vi "Read Temp (SubVI).vi"(8 "error in (no error)":errorcluster, 10 "Channel":string, 11 "Instrument parameters in in":T1) -> (0 "error out":errorcluster, 2 "Sensor Data":dbl, 3 "Instrument parameters out":T1)   [LabVIEW 2025]
uses:
  TYPE DEFS/S2DS_Instrument parameters.ctl
  Lake Shore 336.lvlib
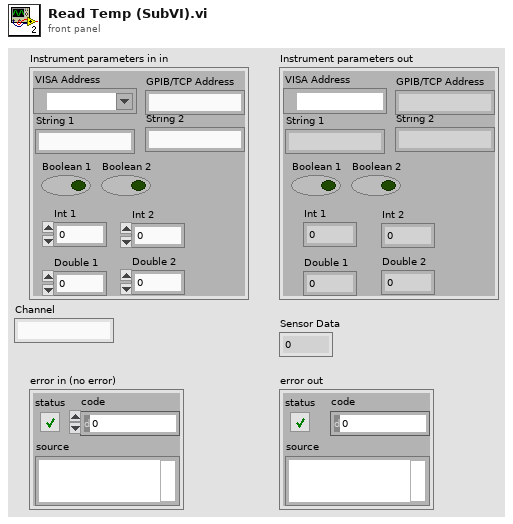
[diagram p1: front panel]
types:
  T1 = typedef "S2DS_Instrument parameters.ctl" = cluster{"VISA Address":refnum<visa-resource-name>, "GPIB/TCP Address":string, "String 1":string, "String 2":string, "Boolean 1":bool, "Boolean 2":bool, "Int 1":i32, "Int 2":i32, "Double 1":dbl, "Double 2":dbl}
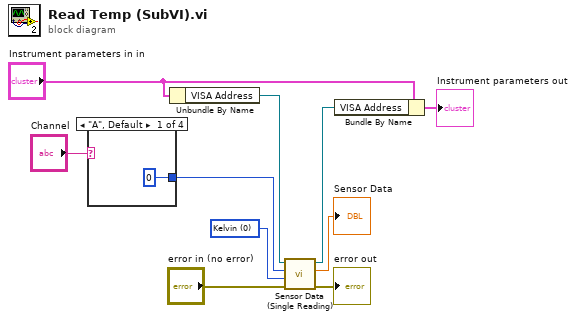
[diagram p0: block diagram]
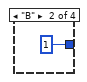
[diagram p2: hidden frame]
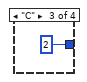
[diagram p3: hidden frame]
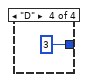
[diagram p4: hidden frame]
diagram:
  w10 = u16 0 items=["Kelvin", "Celsius", "Sensor Units"] ("Data Source (0:Kelvin)")
  n1 = case shown="\"A\", Default" "Channel" {
    tunnel: [0 1 2 3] -> w1
    frame "A", Default {
    }
    frame "B" {
    }
    frame "C" {
    }
    frame "D" {
    }
  }
  n2 = Unbundle By Name("Instrument parameters in in") -> ("VISA Address"=w6:refnum<visa-resource-name>)
  n3 = call "Sensor Data (Single Reading).vi"("error in (no error)"="error in (no error)", "Data Source (0:Kelvin)"=w10, "Input (0:A)"=w1, "VISA resource name"=w6) -> ("error out"=→"error out":errorcluster, "Sensor Data"=→"Sensor Data":dbl, "VISA resource name out"=w5:refnum<visa-resource-name>)  [unwired: 5 in]
  n4 = Bundle By Name(cluster="Instrument parameters in in", "VISA Address"=w5) -> (→"Instrument parameters out":T1)
